vi "Wait for Temperature Setpoint.vi"(4 "Type":enum16{"In Range", "Less", "Greater"}(ring), 6 "Channel":i32, 8 "error in (no error)":errorcluster, 9 "Tolerance (K)":dbl=0.005, 10 "Setpoint (K)":dbl, 11 "Instrument.Cryostat in":refnum<class "Instrument.Cryostat.lvclass">) -> (0 "error out":errorcluster, 3 "Instrument.Cryostat out":refnum<class "Instrument.Cryostat.lvclass">)   [LabVIEW 2019, in "Instrument.Cryostat.lvclass"]
uses:
  Instrument.Cryostat.lvclass
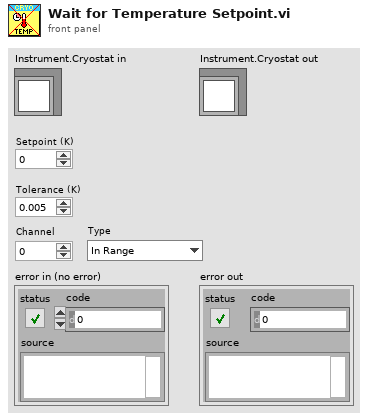
[diagram p1: front panel]
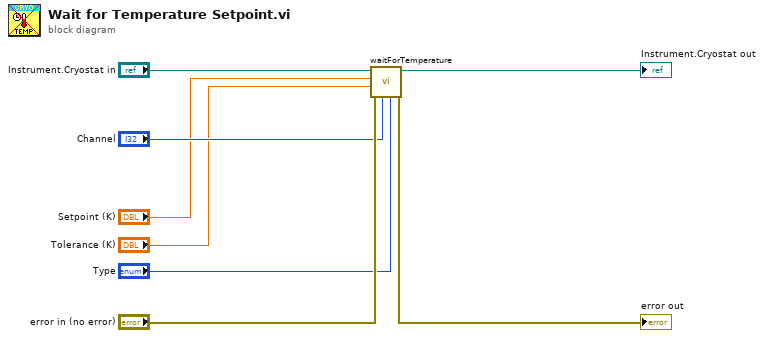
[diagram p0: block diagram]
diagram:
  n1 = call "waitForTemperature.vi"("Type"="Type", "Channel"="Channel", "error in (no error)"="error in (no error)", "Tolerance (K)"="Tolerance (K)", "Setpoint (K)"="Setpoint (K)", "Instrument.Cryostat in"="Instrument.Cryostat in") -> ("error out"=→"error out":errorcluster, "Instrument.Cryostat out"=→"Instrument.Cryostat out":refnum<class "Instrument.Cryostat.lvclass">)  [unwired: 4 in]
